vi "Get Filter.vi"(8 "error in (no error)":errorcluster, 11 "Honeywell Compass HMC6343":refnum<class "Honeywell Compass HMC6343.lvclass">) -> (0 "error out":errorcluster, 2 "Filter":u8, 3 "Honeywell Compass HMC6343 out":refnum<class "Honeywell Compass HMC6343.lvclass">)   [LabVIEW 2019, in "Honeywell Compass HMC6343.lvclass"]
doc: "Gets Filter of the current device."
uses:
  Honeywell Compass HMC6343.lvclass
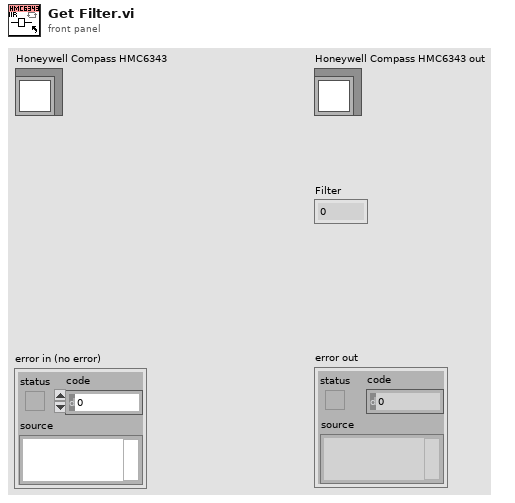
[diagram p1: front panel]
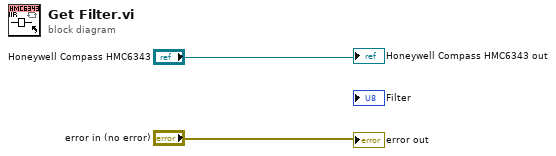
[diagram p0: block diagram]
diagram:
  "error out" <- "error in (no error)"
  "Honeywell Compass HMC6343 out" <- "Honeywell Compass HMC6343"
